vi "Memory.Pointer.Copy.Safe.vi"(8 "error in (no error)":errorcluster, 9 "bytes to copy":u64 format="%08x bytes", 10 "dst pointer in":refnum<class "Memory.Pointer.lvclass">, 11 "src pointer in":refnum<class "Memory.Pointer.lvclass">) -> (0 "error out":errorcluster, 1 "bytes to copy":u64 format="%08x bytes", 2 "dst pointer out":refnum<class "Memory.Pointer.lvclass">, 3 "src pointer out":refnum<class "Memory.Pointer.lvclass">)   [LabVIEW 2016, in "Memory Manager.lvlib" / "Memory.Pointer.lvclass"]
doc: "Copies <b>bytes to copy</b> of data from the memory address specified by <b>src pointer</b> to the memory address specified by <b>dst pointer</b>.\n\n<b>Note:</b> This VI is <b>safe</b>.\n\nSafe means that this function evaluates that the size parameter of <b>dst pointer</b> is greater than or equal to the size of the requested memory from <b>src pointer</b> to ensure that the destination memory location is an appropriate size before copying data from source to destination. Reading/writing more data to a pointer than it has allocated can corrupt or crash LabVIEW."
uses:
  Memory.Pointer.lvclass
  Memory.Pointer.lvclass/Memory.Pointer.ctl
  Accessors/Get Address.vi
  Memory.Pointer.Errors.vi
  Memory.Pointer.Errors.Out of Bounds.vi
  Accessors/Get Size.vi
  Memory.Pointer.Errors.Null Pointer.vi
  Submodules/SEH/Source/VIs/Static Error Handling.Source Buffer.Write.String.vi
  Memory.Pointer.Errors.Write Pointer Size.vi
  Memory.Pointer.Errors.Create Error.vi
  Submodules/SEH/Source/VIs/Static Error Handling.Source Buffer.Write.Numeric.Scalar.Base10.vi
  Submodules/SEH/Source/VIs/Static Error Handling.Source Buffer.Write.Numeric.Scalar.Base10 (U64).vi
  Submodules/SEH/Source/VIs/Static Error Handling.Error Cluster Constant.vi
  Submodules/SEH/Source/VIs/Static Error Handling.Error Cluster Constant (256B).vi
  Submodules/SEH/Source/VIs/Static Error Handling.Parameters.Status.Set.vi
  Submodules/SEH/Source/VIs/Static Error Handling.Parameters.Code.Set.vi
  Submodules/SEH/Source/VIs/Static Error Handling.Parameters.VI Source.Set.vi
  Constants/Memory.Constants.vi
  Constants/Memory.Constants.Library Name.vi
  Memory.Pointer.Errors.Get Info.vi
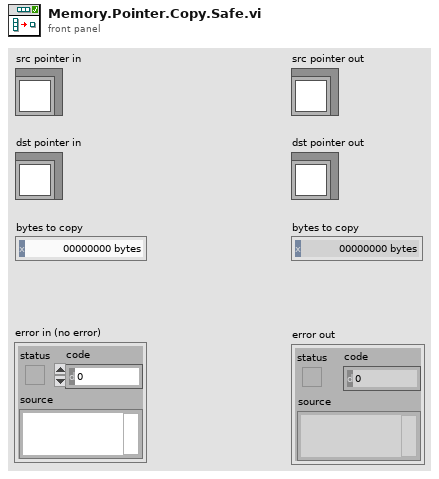
[diagram p1: front panel]
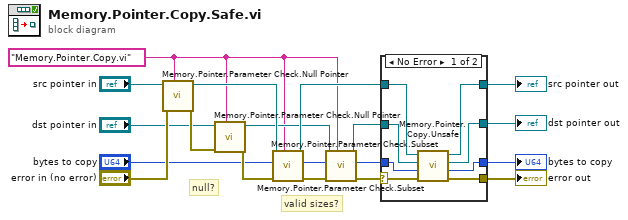
[diagram p0: block diagram]
diagram:
  w4 = "Memory.Pointer.Copy.vi" ("source vi name")
  # "valid sizes?"
  # "null?"
  n1 = call "Memory.Pointer.Parameter Check.Null Pointer.vi"("source vi name"=w4, "error in (no error)"="error in (no error)", "Pointer in"="src pointer in") -> ("error out"=w8:errorcluster, "Pointer out"=w10:refnum<class "Memory.Pointer.lvclass">)  [unwired: 7 in]
  n2 = call "Memory.Pointer.Parameter Check.Null Pointer.vi"("source vi name"=w4, "error in (no error)"=w8, "Pointer in"="dst pointer in") -> ("error out"=w6:errorcluster, "Pointer out"=w9:refnum<class "Memory.Pointer.lvclass">)  [unwired: 7 in]
  n3 = call "Memory.Pointer.Parameter Check.Subset.vi"("source vi name"=w4, "error in (no error)"=w6, "length"="bytes to copy", "Pointer in"=w10) -> ("error out"=w15:errorcluster, "length"=w3:u64, "Pointer out"=w13:refnum<class "Memory.Pointer.lvclass">)  [unwired: 4 in, 1 out]
  n4 = call "Memory.Pointer.Parameter Check.Subset.vi"("source vi name"=w4, "error in (no error)"=w15, "length"=w3, "Pointer in"=w9) -> ("error out"=w14:errorcluster, "length"=w2:u64, "Pointer out"=w12:refnum<class "Memory.Pointer.lvclass">)  [unwired: 4 in, 1 out]
  n5 = case shown="No Error" w14 {
    selector: w14 -> [w20 w28]
    tunnel: [w24 w29] -> w19
    tunnel: w2 -> [w25 w29]
    tunnel: w13 -> [w27 w31]
    tunnel: w12 -> [w26 w30]
    tunnel: [w22 w31] -> w18
    tunnel: [w21 w30] -> w17
    tunnel: [w23 w28] -> w16
    frame No Error {
      n6 = call "Memory.Pointer.Copy.Unsafe.vi"("error in (no error)"=w20, "bytes to copy"=w25, "dst pointer in"=w26, "src pointer in"=w27) -> ("error out"=w23:errorcluster, "bytes to copy"=w24:u64, "dst pointer out"=w21:refnum<class "Memory.Pointer.lvclass">, "src pointer out"=w22:refnum<class "Memory.Pointer.lvclass">)  [unwired: 4 in]
    }
    frame Error {
    }
  }
  "error out" <- w16
  "src pointer out" <- w18
  "dst pointer out" <- w17
  "bytes to copy" <- w19
